vi "Read Temperature Range.vi"(8 "error in (no error)":errorcluster, 11 "Cooler in":refnum<class "Cooler.lvclass">) -> (0 "error out":errorcluster, 1 "Max Temp":dbl, 2 "Min Temp":dbl, 3 "Cooler out":refnum<class "Cooler.lvclass">)   [LabVIEW 2018, in "Cooler.lvclass"]
uses:
  Cooler.lvclass
  Cooler.lvclass/Cooler.ctl
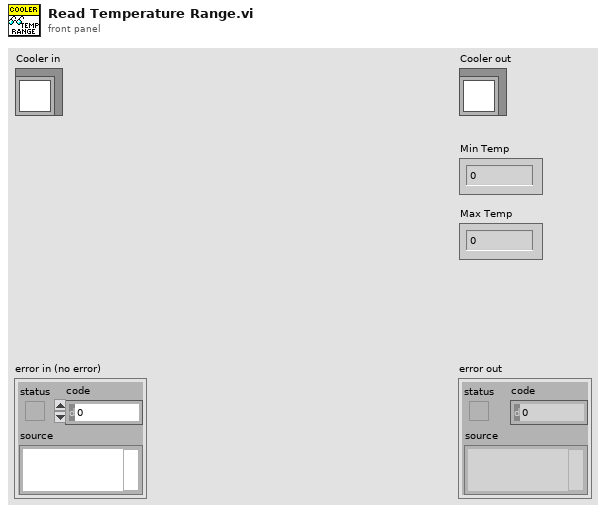
[diagram p1: front panel]
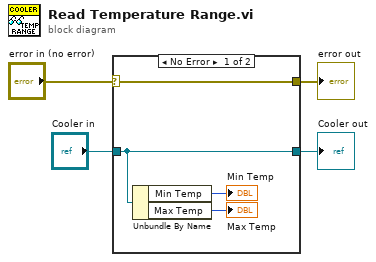
[diagram p0: block diagram]
diagram:
  n1 = case shown="No Error" "error in (no error)" {
    selector: "error in (no error)" -> [w8 w9]
    tunnel: [w8 w9] -> w3
    tunnel: [w7 w10] -> w1
    tunnel: "Cooler in" -> [w7 w10]
    frame No Error {
      n2 = Unbundle By Name(w7) -> ("Min Temp"=→"Min Temp":i32, "Max Temp"=→"Max Temp":i32)
    }
    frame Error {
    }
  }
  "error out" <- w3
  "Cooler out" <- w1
